vi "SRV_Sensor Caption Text.vi"(5 "Name":string, 9 "Units":string) -> (8 "Sensor Caption Text":string)   [LabVIEW 2009]
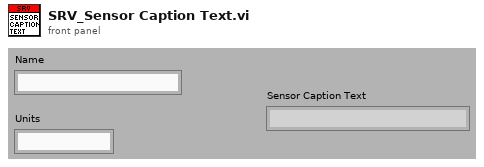
[diagram p1: front panel]
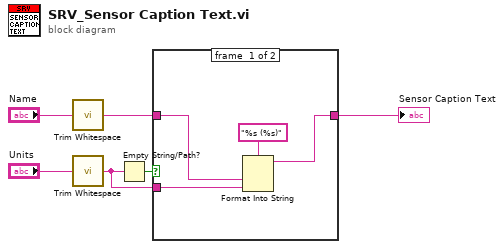
[diagram p0: block diagram]
diagram:
  n1 = call <vilib>:"Trim Whitespace.vi"("string"="Name") -> ("trimmed string"=w3:string)  [unwired: 1 in]
  n2 = call <vilib>:"Trim Whitespace.vi"("string"="Units") -> ("trimmed string"=w1:string)  [unwired: 1 in]
  n3 = Empty String/Path?(string/path=w1) -> (empty?=w4:bool)
  n4 = case shown="False" w4 {
    tunnel: w3 -> [w9 w11]
    tunnel: [w7 w11] -> w2
    tunnel: w1 -> [w8 _]
    frame #0 {
      n5 = Format Into String(format string="%s (%s)", w9, w8) -> (resulting string=w7:string)  [unwired: 2 in, 1 out]
    }
    frame #1 {
    }
  }
  "Sensor Caption Text" <- w2
